vi "XY Zto RGB24.vi"(8 "error in (no error)":errorcluster, 10 "para1":cluster{}, 11 "para0":cluster{}) -> (0 "error out":errorcluster, 1 "function return":u32, 2 "para1 out":cluster{}, 3 "para0 out":cluster{})   [LabVIEW 2018]
doc: "LIBTIFF_DLL_IMPEXP void XYZtoRGB24(float*, uint8*);\nextern void XYZtoRGB24(float*, uint8*);"
uses:
  libtiff3.dll
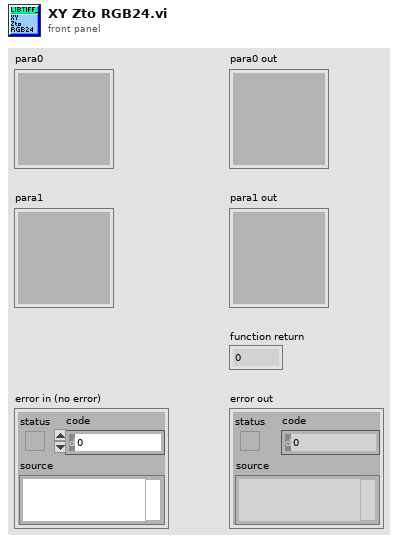
[diagram p1: front panel]
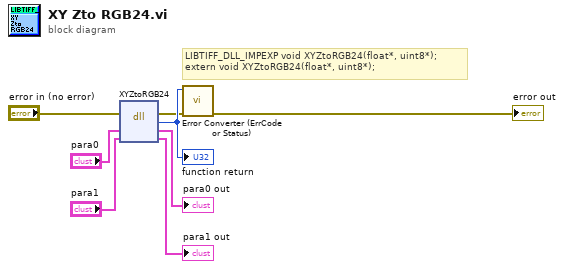
[diagram p0: block diagram]
diagram:
  # "LIBTIFF_DLL_IMPEXP\tvoid XYZtoRGB24(float*, uint8*);\nextern\tvoid XYZtoRGB24(float*, uint8*);"
  n1 = dll-call lib="C:/Users/johan/Downloads/LabVIEW software/LabVIEW software/IX-81 Software/lib/tiff/LibTiffLabview/libtiff3.*" fn="XYZtoRGB24"(error in="error in (no error)", "para0"="para0", "para1"="para1") -> (error out=w2:errorcluster, w8:u32, "para0"=→"para0 out":cluster{}, "para1"=→"para1 out":cluster{})  [unwired: 2 in, 1 out]
  "function return" <- w8
  n2 = call "Error Converter (ErrCode or Status).vi"("error in (no error)"=w2, "error code"=w8) -> ("error out"=→"error out":errorcluster)  [unwired: 9 in]
